vi "SwerveKinematics_ToChassisSpeeds4.vi"(7 "in SWERVE_DRIVE_KINEMATICS":T4 {"PrevCoR"."Y" format="%14.3f"; "PrevCoR"."X" format="%14.3f"; "Modules"."Y" format="%14.3f"; "Modules"."X" format="%14.3f"}, 8 "Wheel State 3":T1={"Speed"=0.0, "Angle"={"VALUE"=0.0, "COS"=1.0, "SIN"=0.0}} {"Angle"."SIN" format="%13.4f"; "Angle"."COS" format="%13.4f"; "Angle"."VALUE" format="%13.4f"}, 9 "Wheel State 2":T1={"Speed"=0.0, "Angle"={"VALUE"=0.0, "COS"=1.0, "SIN"=0.0}} {"Angle"."SIN" format="%13.4f"; "Angle"."COS" format="%13.4f"; "Angle"."VALUE" format="%13.4f"}, 10 "Wheel State 1":T1={"Speed"=0.0, "Angle"={"VALUE"=0.0, "COS"=1.0, "SIN"=0.0}} {"Angle"."SIN" format="%13.4f"; "Angle"."COS" format="%13.4f"; "Angle"."VALUE" format="%13.4f"}, 11 "Wheel State 0":T1={"Speed"=0.0, "Angle"={"VALUE"=0.0, "COS"=1.0, "SIN"=0.0}} {"Angle"."SIN" format="%13.4f"; "Angle"."COS" format="%13.4f"; "Angle"."VALUE" format="%13.4f"}) -> (1 "Chassis Speed":T3)   [LabVIEW 2019, in "Trajectory_Library.lvlib"]
doc: "Performs forward kinematics to return the resulting chassis state from the given module states. This method is often used for odometry -- determining the robot's position on the field using data from the real-world speed and angle of each module on the robot. This subVI is customized for 4 individual wheel states.\n\nParameters: \n - in Swerve Drive Kinematics - Swerve drive kinematics data structure\n - wheelState 0 - The state of a module (as a SwerveModuleState type) as measured from respective encoders and gyros. The order of the swerve module states should be same as passed into the constructor of this class.\n - wheelState 1 - Another wheel state \n - wheelState 2 - Another wheel state\n - wheelState 3 - Another wheel state\n\nReturns:\n - The resulting chassis speed."
uses:
  Trajectory_Library.lvlib
  SWERVE_DRIVE_KINEMATICS.ctl
  <vilib>/Analysis/Matrix/Datatypes/RealMatrix.ctl
  TRANSLATION2D.ctl
  CHASSIS_SPEEDS.ctl
  SWERVE_DRIVE_MODULE_STATE.ctl
  ROTATION2D.ctl
  <vilib>/Analysis/Matrix/NI_Matrix.lvlib
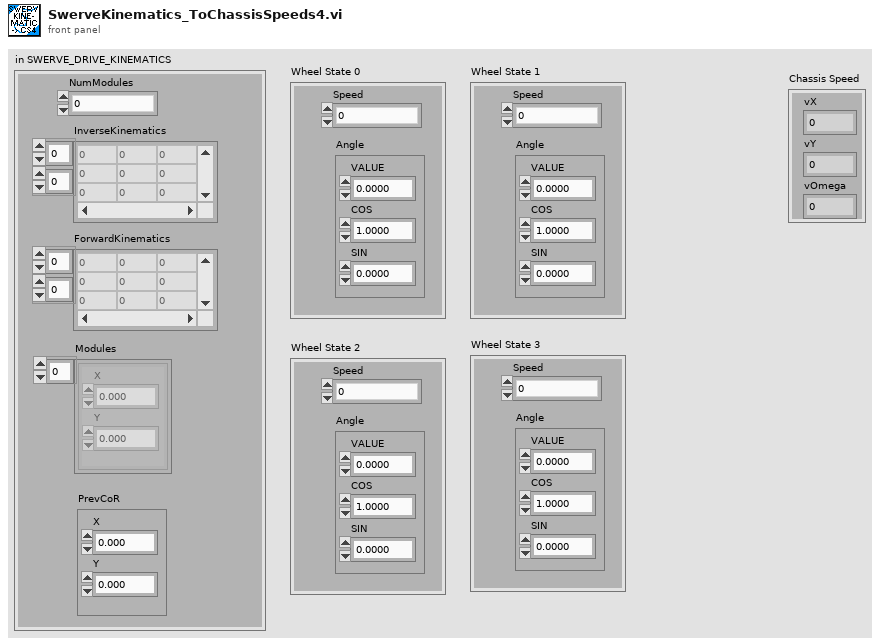
[diagram p1: front panel]
types:
  T1 = typedef "Trajectory_Library.lvlib/SWERVE_DRIVE_MODULE_STATE.ctl" = cluster{"Speed":dbl, "Angle":T2}
  T2 = typedef "Trajectory_Library.lvlib/ROTATION2D.ctl" = cluster{"VALUE":dbl, "COS":dbl, "SIN":dbl}
  T3 = typedef "Trajectory_Library.lvlib/CHASSIS_SPEEDS.ctl" = cluster{"vX":dbl, "vY":dbl, "vOmega":dbl}
  T4 = typedef "Trajectory_Library.lvlib/SWERVE_DRIVE_KINEMATICS.ctl" = cluster{"NumModules":i32, "InverseKinematics":T5, "ForwardKinematics":T5, "Modules":T6[], "PrevCoR":T6}
  T5 = typedef "NI_Matrix.lvlib/RealMatrix.ctl" = dbl[][]
  T6 = typedef "Trajectory_Library.lvlib/TRANSLATION2D.ctl" = cluster{"X":dbl, "Y":dbl}
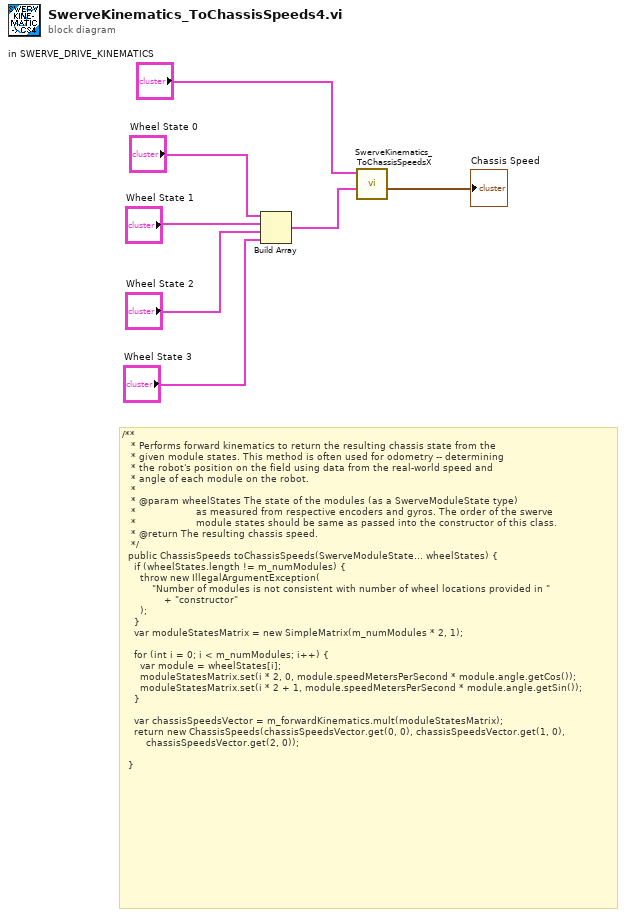
[diagram p0: block diagram]
diagram:
  # "/**\n   * Performs forward kinematics to return the resulting chassis state from the\n   * given module states. This method is often used for odometry -- determining\n   * the robot's position on the field using data from the real-world speed and\n   * angle of each module on the robot.\n   *\n   * @param wheelStates The state of the modules (as a SwerveModuleState type)\n   *                    as measured from respective encoders and gyros. The order of the swerve\n   *                    module states should be same as passed into the constructor of this class.\n   * @return The resulting chassis speed.\n   */\n  public ChassisSpeeds toChassisSpeeds(SwerveModuleState... wheelStates) {\n    if (wheelStates.length != m_numModules) {\n      throw new IllegalArgumentException(\n          \"Number of modules is not consistent with number of wheel locations provided in \"\n              + \"constructor\"\n      );\n    }\n    var moduleStatesMatrix = new SimpleMatrix(m_numModules * 2, 1);\n\n    for (int i = 0; i < m_numModules; i++) {\n      var module = wheelStates[i];\n      moduleStatesMatrix.set(i * 2, 0, module.speedMetersPerSecond * module.angle.getCos());\n      moduleStatesMatrix.set(i * 2 + 1, module.speedMetersPerSecond * module.angle.getSin());\n    }\n\n    var chassisSpeedsVector = m_forwardKinematics.mult(moduleStatesMatrix);\n    return new ChassisSpeeds(chassisSpeedsVector.get(0, 0), chassisSpeedsVector.get(1, 0),\n        chassisSpeedsVector.get(2, 0));\n\n  }"
  n1 = Build Array("Wheel State 0", "Wheel State 1", "Wheel State 2", "Wheel State 3") -> (w2:T1[])
  n2 = call "SwerveKinematics_ToChassisSpeedsX.vi"("WheelStates"=w2, "in SWERVE_DRIVE_KINEMATICS"="in SWERVE_DRIVE_KINEMATICS") -> ("Chassis Speed"=→"Chassis Speed":T3)  [unwired: 9 in]
